vi "RunSuite.vi"(11 "Command Line Args":string[](array[string])) -> (2 "Return Message":string="No Error", 3 "Return Code":i32)   [LabVIEW 2016]
uses:
  <vilib>/Utility/error.llb/DialogType.ctl
  <vilib>/addons/_JKI Toolkits/Caraya/classes/Test Suite/Define Test Suite (JUnit Report).vi
  <vilib>/addons/_JKI Toolkits/Caraya/classes/Test Suite/Test Suite.lvclass
panel:
  in  "Interactive":bool
  # "Can specify report path as first argument"
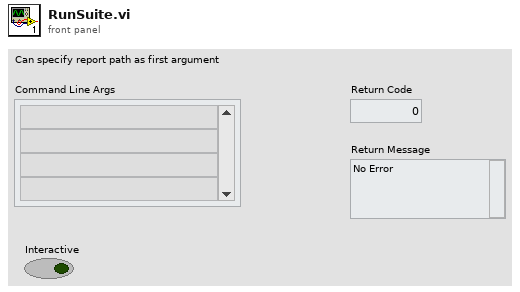
[diagram p1: front panel]
types:
  T1 = typedef "DialogType.ctl" = u16
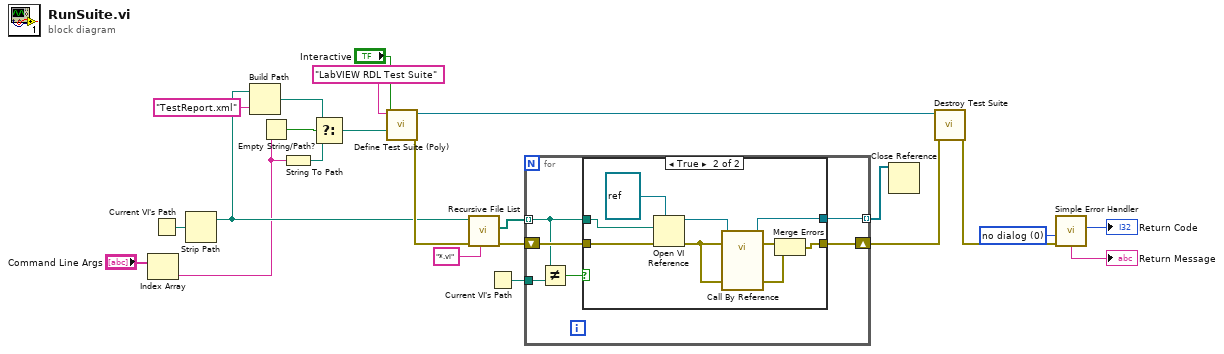
[diagram p0: block diagram]
diagram:
  w14 = T1 0 items=["no dialog", "OK message", "continue or stop message", "OK message + warnings", "continue/stop + warnings"] ("type of dialog (OK msg:1)")
  n1 = Index Array(array="Command Line Args") -> (element=w3:string)  [unwired: 1 in]
  n2 = Current VI's Path() -> (path=w23:path)
  n3 = Strip Path(path=w23) -> (stripped path=w9:path)  [unwired: 1 out]
  n4 = Build Path(base path=w9, name or relative path="TestReport.xml") -> (appended path=w10:path)
  n5 = Empty String/Path?(string/path=w3) -> (empty?=w2:bool)
  n6 = String To Path(string=w3) -> (path=w6:path)
  n7 = Select(t=w10, s=w2, f=w6) -> (s? t:f=w7:path)
  n8 = call-poly <vilib>:"Define Test Suite (Poly).vi"("Report Path"=w7, "Interactive"="Interactive", "Label (VI Title)"="LabVIEW RDL Test Suite") -> ("error out"=w20:errorcluster, "Test Suite"=w21:refnum<class "Test Suite.lvclass">)  [unwired: 7 in]
  n9 = call <vilib>:"Recursive File List.vi"("pattern"="*.vi", "error in (no error)"=w20, "Folder Path"=w9) -> ("error out"=w19:errorcluster, "All Files in Dir"=w5:path[])  [unwired: 4 in, 3 out]
  n10 = Current VI's Path() -> (path=w4:path)
  n11 = for {
    tunnel: w5 -> [w26] mode=indexing
    shift-right: [w28] -> w17
    shift-left: w19 -> [w29]
    tunnel: [w27] -> w16 mode=indexing
    tunnel: w4 -> [w25]
    n12 = Not Equal?(x=w26, y=w25) -> (x != y?=w24:bool)
    n13 = case shown="True" w24 {
      tunnel: w29 -> [w30 w39]
      tunnel: w26 -> [_ w38]
      tunnel: [w30 w32] -> w28
      tunnel: [_ w36] -> w27
      frame False {
        # "Don't run the current VI!"
      }
      frame True {
        n14 = Open VI Reference(type specifier VI Refnum (for type only)=refnum<vi> refnum, vi path=w38, error in (no error)=w39) -> (vi reference=w34:refnum<vi>, error out=w33:errorcluster)  [unwired: 3 in]
        n15 = call-by-ref "?"(reference=w34, error in=w33, 8:"error in (no error)"=w33) -> (reference out=w36:refnum<vi>, error out=w37:errorcluster, 0:"error out"=w31:errorcluster)  [unwired: 10 in]
        n16 = Merge Errors(w37, w31) -> (w32:errorcluster)
      }
    }
  }
  n17 = Close Reference(reference=w16) -> ()  [unwired: 1 in, 1 out]
  n18 = call-dynamic "Destroy Test Suite.vi"("error in (no error)"=w17, "Test Suite in"=w21) -> ("error out"=w15:errorcluster)  [unwired: 9 in]
  n19 = call <vilib>:"Simple Error Handler.vi"("type of dialog (OK msg:1)"=w14, "error in (no error)"=w15) -> ("code out"=→"Return Code":i32, "message"=→"Return Message":string)  [unwired: 3 in, 3 out]
